vi "PrefDialog.vi"(8 "error in (no error)":errorcluster, 11 "MyPluginsBase in":refnum<class "NHRDCModel.lvclass">) -> (0 "error out":errorcluster, 1 "Save As":bool, 2 "Changed":bool, 3 "MyPluginsBase out":refnum<class "NHRDCModel.lvclass">)   [LabVIEW 2018, in "AcPwrPlugins.lvlib" / "NHRDCModel.lvclass"]
doc: "This VI displays the prior instruments properties and allows a user to change the instrument properties and save these new set properties to the same location on disk or in a new location with a new name called \"Type\"."
uses:
  NHRDCModel.lvclass
  <vilib>/Utility/config.llb/NI_LVConfig.lvlib
  AcPwrBaseClass/AcPwrBase.lvclass
  NHRDCPowerClass/TypeDefs/Modules.ctl
  NHRDCPowerClass/NHRDCPower.lvclass
  NHRDCPowerClass/TypeDefs/Device(s)Settings.ctl
  NHRDCPowerClass/TypeDefs/Measurements.ctl
panel:
  in  "btnSaveAs":bool
  in  "btnSave":bool
  in  "Measurement RefreshTime (ms)":u32
  in  "btnCancel":bool
  in  "Measurements":T1
  in  "Device(s)Settings":T2 {"Modules"."Regulation Gain (1=100%)" min=0.0 max=1.0; "Modules"."OutputSettings"."Wait on Value" items=["Voltage Greater Than Or Equal To", "Voltage Less Than Or Equal To", "Current Greater Than Or Equal To", "Current Less Than Or Equal To", "Power Greater Than Or Equal To", "Power Less Than Or Equal To"]; "Modules"."operating state (Off)" items=["Off", "Stand By", "Charge", "Discharge", "Battery Emulation"]}
  # "*Please ensure that Voltage and Current are selected as the 1st and 2nd Measurement variables, respectively, to correctly plot Voltage vs Current in the visualization VI."
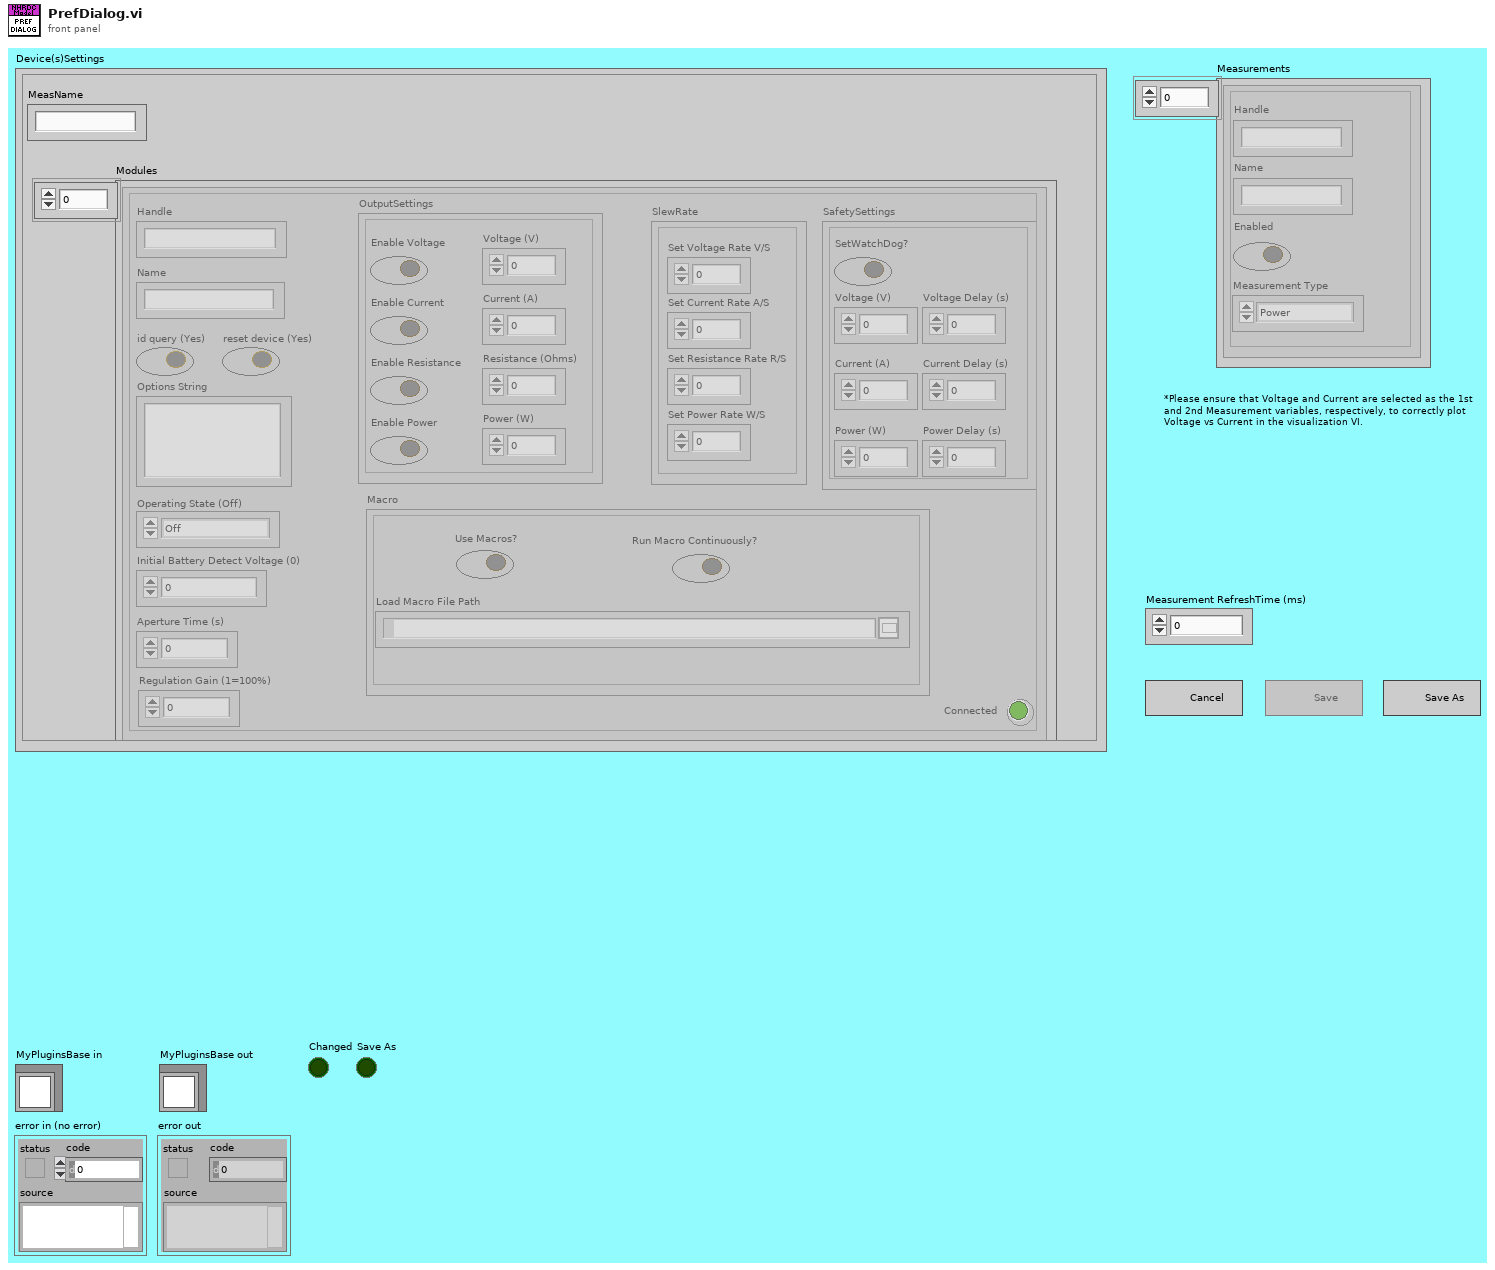
[diagram p1: front panel]
types:
  T1 = typedef "AcPwrPlugins.lvlib/NHRDCPower.lvclass/Measurements.ctl" = cluster{"Handle":string, "Name":string, "Enabled":bool, "Measurement Value":sgl, "Measurement Type":enum16{"Power", "Current", "Voltage"}}[]
  T2 = typedef "AcPwrPlugins.lvlib/NHRDCPower.lvclass/Device(s)Settings.ctl" = cluster{"MeasName":string, "Modules":T3}
  T3 = typedef "AcPwrPlugins.lvlib/NHRDCPower.lvclass/Modules.ctl" = cluster{"Handle":string, "Name":string, "id query (Yes)":bool, "reset device (Yes)":bool, "Connected":bool, "Initial Battery Detect Voltage (0)":dbl, "SafetySettings":cluster{"SetWatchDog?":bool, "Voltage (V)":dbl, "Current (A)":dbl, "Power (W)":dbl, "Voltage Delay (s)":dbl, "Current Delay (s)":dbl, "Power Delay (s)":dbl}, "Options String":string, "Aperture Time (s)":dbl, "operating state (Off)":i32, "OutputSettings":cluster{"Voltage (V)":dbl, "Current (A)":dbl, "Resistance (Ohms)":dbl, "Power (W)":dbl, "Enable Voltage":bool, "Enable Current":bool, "Enable Resistance":bool, "Enable Power":bool, "Macro After Step Delay  (s)":dbl, "Wait Value (V, A, W)":dbl, "Enable Wait":bool, "Wait on Value":i32}, "SlewRate":cluster{"Set Voltage Rate V/S":dbl, "Set Current Rate A/S":dbl, "Set Resistance Rate R/S":dbl, "Set Power Rate W/S":dbl}, "Macro":cluster{"Save Macro?":bool, "Load Macro From File?":bool, "Run Macro Continuously?":bool, "Use Macros?":bool, "Load Macro File Path":path, "Save Macro File Path":string}, "Regulation Gain (1=100%)":dbl, "UpdatingOntheFly":bool}[]
  T4 = enum8{"Enabled", "Disabled", "Disabled and Grayed Out"}
  T5 = enum32{"Invalid", "Default", "Floating", "Floating/Auto-Hide", "Modal"}
  T6 = cluster{"Handle":string, "Name":string, "id query (Yes)":bool, "reset device (Yes)":bool, "Connected":bool, "Initial Battery Detect Voltage (0)":dbl, "SafetySettings":cluster{"SetWatchDog?":bool, "Voltage (V)":dbl, "Current (A)":dbl, "Power (W)":dbl, "Voltage Delay (s)":dbl, "Current Delay (s)":dbl, "Power Delay (s)":dbl}, "Options String":string, "Aperture Time (s)":dbl, "operating state (Off)":i32, "OutputSettings":cluster{"Voltage (V)":dbl, "Current (A)":dbl, "Resistance (Ohms)":dbl, "Power (W)":dbl, "Enable Voltage":bool, "Enable Current":bool, "Enable Resistance":bool, "Enable Power":bool, "Macro After Step Delay  (s)":dbl, "Wait Value (V, A, W)":dbl, "Enable Wait":bool, "Wait on Value":i32}, "SlewRate":cluster{"Set Voltage Rate V/S":dbl, "Set Current Rate A/S":dbl, "Set Resistance Rate R/S":dbl, "Set Power Rate W/S":dbl}, "Macro":cluster{"Save Macro?":bool, "Load Macro From File?":bool, "Run Macro Continuously?":bool, "Use Macros?":bool, "Load Macro File Path":path, "Save Macro File Path":string}, "Regulation Gain (1=100%)":dbl, "UpdatingOntheFly":bool}
  T7 = typedef "AcPwrPlugins.lvlib/AcPwrBase.lvclass/BaseConfig.ctl" = cluster{"Frequency":dbl, "FrequencyRange":dbl[], "Phases":T8[], "Name":string, "PluginConfigVariant":variant, "PluginMeasVariant":variant}
  T8 = typedef "AcPwrPlugins.lvlib/AcPwrBase.lvclass/Phase.ctl" = cluster{"Name":string, "Enabled":bool, "VoltageLevel":dbl, "Handle":string, "VoltageRange":dbl[], "Connected":bool, "CurrentLimit":dbl, "Waveform":string}
  T9 = typedef "AcPwrPlugins.lvlib/AcPwrBase.lvclass/BaseMeasurements.ctl" = cluster{"Handle":string, "Name":string, "Enabled":bool, "Measurement Value":dbl, "btnMeasFetch":bool, "Chroma Hold Peak Current Measurement":bool, "Chroma Measurement Type":T10, "Chroma Protection Status String":string, "NHRDC Fetch Method":i32, "NHRDC Fetch Time (s)":sgl, "NHRDC Measurement Type":i32, "NHRGridSim Measurement Type ":enum16{"Average Current", "Max Current", "Min Current", "Average Voltage", "Max Voltage", "Min Voltage", "Average True Power", "Max True Power", "Min True Power", "Average Apparent Power", "Max Apparent Power", "Min Apparent Power", "Power Factor", "Crest Factor"}, "NHRGridSim Phase ":i32, "PPS Measurement Type ":enum16{"Voltage RMS L-N", "Voltage RMS L-L", "Frequency", "Current RMS", "Current Peak", "Crest Factor", "Power Factor", "Power VA", "Real Power"}, "PPS Channel Name":enum16{"A", "B", "C"}}[]
  T10 = typedef "AcPwrPlugins.lvlib/ChromaAcLoad.lvclass/MeasurementType.ctl" = enum16{"Voltage (Vrms or V)", "Current (Arms or A)", "Power (W)", "Peak Voltage (V)", "Peak Current (A)", "Peak Power (W)", "Frequency (Hz)", "Resistance (Ohms)", "Voltage Overshoot (V)", "Positive Peak Current (A)", "Voltage Undershoot (V)", "Negative Peak Current (A)", "Apparent Power (VA)", "Reacitive Power (VAR)", "Voltage THD", "Power Factor", "Current's Crest Factor"}
  T11 = typedef "NI_LVConfig.lvlib/Config Data RefNum.ctl" = refnum<k1>
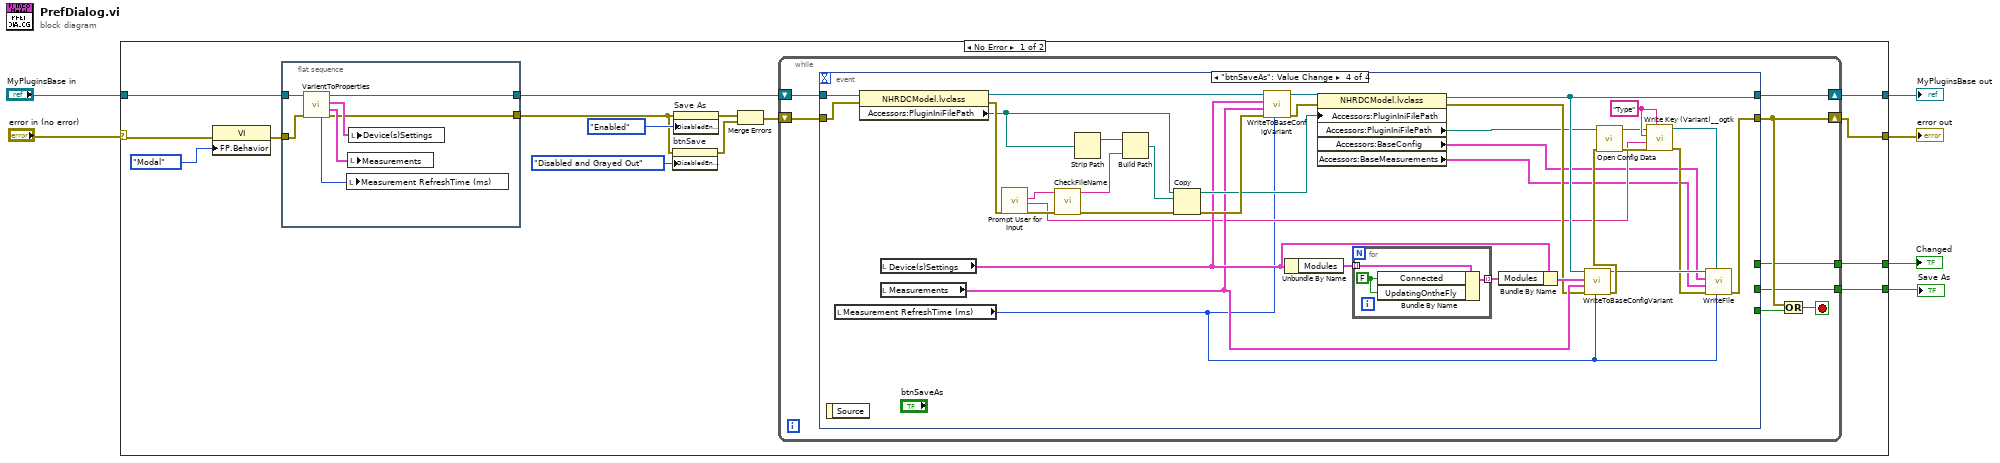
[diagram p0: block diagram]
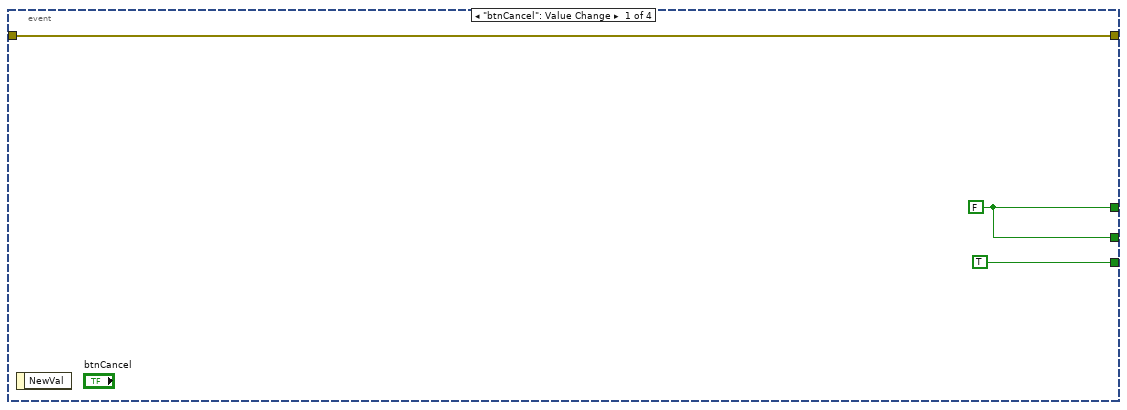
[diagram p2: hidden frame]
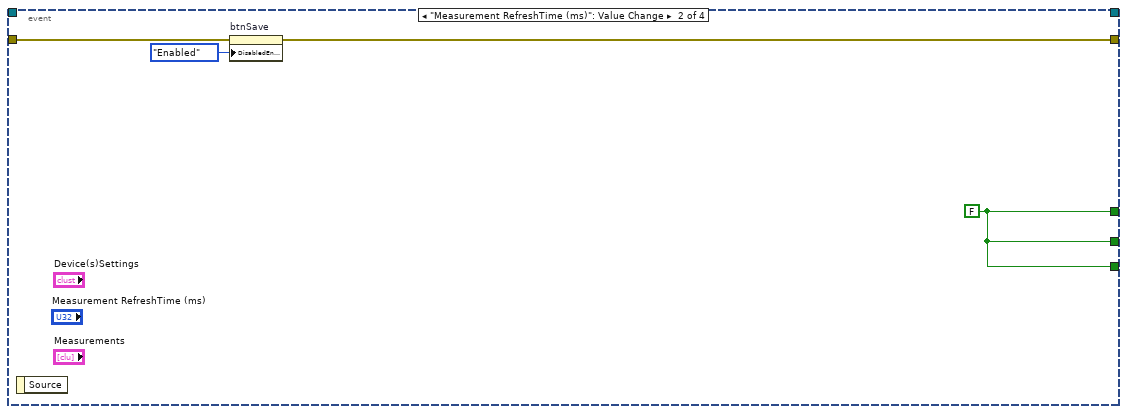
[diagram p3: hidden frame]
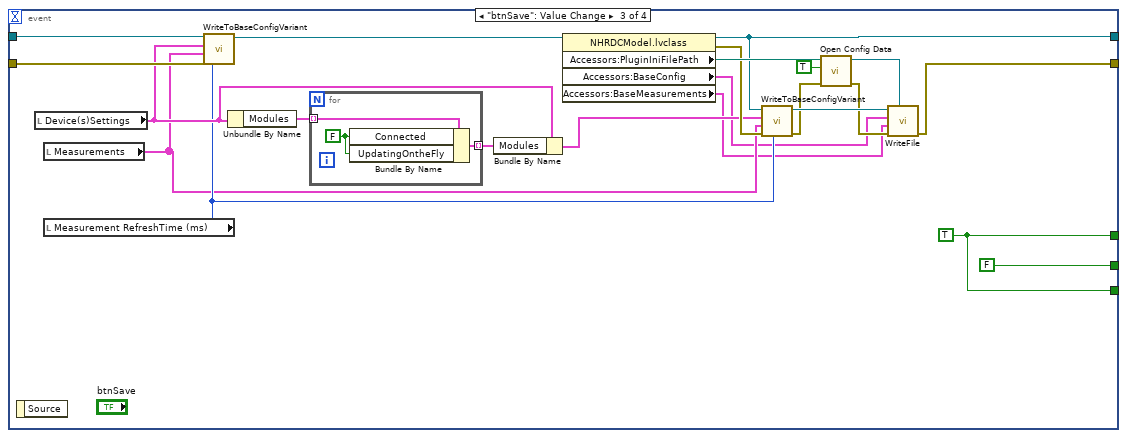
[diagram p4: hidden frame]
diagram:
  n1 = case shown="No Error" "error in (no error)" {
    selector: "error in (no error)" -> [w20 w107]
    tunnel: "MyPluginsBase in" -> [w19 w108]
    tunnel: [w10 w108] -> w4
    tunnel: [w9 w107] -> w3
    tunnel: [w8 _] -> w2
    tunnel: [w7 _] -> w1
    frame No Error {
      n2 = property class="VI"(error in=w20, "FP.Behavior"=T5."Modal" ("Front Panel Window:Behavior")) -> (error out=w18:errorcluster)  [unwired: 1 in, 1 out]
      n3 = flat-sequence {
        tunnel: w19 -> [w106]
        tunnel: w18 -> [w105]
        tunnel: [w101] -> w12
        tunnel: [w100] -> w16
        frame #0 {
          n4 = call "VarientToProperties.vi"("error in (no error)"=w105, "AcPwrPlugins.lvlib:NHRDCModel.lvclass"=w106) -> ("error out"=w100:errorcluster, "Measurements"=w103:T1, "Device(s)Settings"=w104:T2, "AcPwrPlugins.lvlib:NHRDCModel.lvclass"=w101:refnum<class "NHRDCModel.lvclass">, "Measurement Refresh Time (ms)"=w102:u32)  [unwired: 4 in, 1 out]
          n5 = local write "Measurement RefreshTime (ms)"(w102) -> ()
          n6 = local write "Measurements"(w103) -> ()
          n7 = local write "Device(s)Settings"(w104) -> ()
        }
      }
      n8 = property on="btnSave" class="Bool"(error in=w16, "DisabledEnum"=T4."Disabled and Grayed Out" ("Disabled")) -> (error out=w13:errorcluster)  [unwired: 1 in, 1 out]
      n9 = property on="Save As" class="Bool (strict)"(error in=w16, "DisabledEnum"=T4."Enabled" ("Disabled")) -> (error out=w14:errorcluster)  [unwired: 1 in, 1 out]
      n10 = Merge Errors(w14, w13) -> (w11:errorcluster)
      n11 = while {
        shift-right: [w24] -> w10
        shift-left: w12 -> [w29]
        shift-right: [w25] -> w9
        shift-left: w11 -> [w28]
        tunnel: [w23] -> w8
        tunnel: [w22] -> w7
        stop <- w26 stop-if-true
        n12 = event shown="[3] \"btnSaveAs\": Value Change" {
          selector: _ -> [_ _ _ _]
          dyn-events: _ -> [_ _ _ _]
          timeout: _ -> [_ _ _ _]
          tunnel: w29 -> [_ _ w58 w96]
          tunnel: w28 -> [w32 w36 w57 w95]
          tunnel: [w32 w34 w39 w65] -> w25
          tunnel: [TRUE w33 w37 _] -> w27
          tunnel: [w30 w33 w37 _] -> w23
          tunnel: [w30 w33 FALSE _] -> w22
          tunnel: [_ _ w50 w79] -> w24
          event "btnCancel": Value Change {
            w30 = FALSE
            n13 = event-data() -> ()  [unwired: 1 in, 1 out]
          }
          event "Measurement RefreshTime (ms)": Value Change {
            w33 = FALSE
            n14 = event-data() -> ()  [unwired: 1 in, 1 out]
            n15 = property on="btnSave" class="Bool"(error in=w36, "DisabledEnum"=T4."Enabled" ("Disabled")) -> (error out=w34:errorcluster)  [unwired: 1 in, 1 out]
          }
          event "btnSave": Value Change {
            w37 = TRUE
            n16 = event-data() -> ()  [unwired: 1 in, 1 out]
            n17 = local read "Device(s)Settings"() -> (w55:T2)
            n18 = local read "Measurements"() -> (w46:T1)
            n19 = local read "Measurement RefreshTime (ms)"() -> (w48:u32)
            n20 = call-dynamic "WriteToBaseConfigVariant.vi"("Measurement Refresh Time (ms)"=w48, "error in (no error)"=w57, "Meas"=w46, "Config"=w55, "NHRDCModel in"=w58) -> ("NHRDCModel out"=w53:refnum<class "NHRDCModel.lvclass">)  [unwired: 5 in, 1 out]
            n21 = Unbundle By Name(w55) -> ("Modules"=w56:T3)
            n22 = for {
              tunnel: w56 -> [w61] mode=indexing
              tunnel: [w59] -> w54 mode=indexing
              w60 = FALSE ("Connected")
              n23 = Bundle By Name(cluster=w61, "Connected"=w60, "UpdatingOntheFly"=w60) -> (w59:T6)
            }
            n24 = Bundle By Name(cluster=w55, "Modules"=w54) -> (w47:T2)
            n25 = property class="NHRDCModel.lvclass"(reference=w53) -> (reference out=w50:refnum<class "NHRDCModel.lvclass">, error out=w49:errorcluster, "Accessors:PluginIniFilePath"=w52:path, "Accessors:BaseConfig"=w41:T7, "Accessors:BaseMeasurements"=w40:T9)  [unwired: 1 in]
            n26 = call-dynamic "WriteToBaseConfigVariant.vi"("Measurement Refresh Time (ms)"=w48, "error in (no error)"=w49, "Meas"=w46, "Config"=w47, "NHRDCModel in"=w50) -> ("error out"=w44:errorcluster, "NHRDCModel out"=w45:refnum<class "NHRDCModel.lvclass">)  [unwired: 5 in]
            n27 = call <vilib>:"Open Config Data.vi"("error in (no error)"=w44, "create file if necessary (T)"=TRUE, "configuration file path"=w52) -> ("error out"=w43:errorcluster, "refnum"=w42:T11)  [unwired: 6 in, 1 out]
            n28 = call-dynamic "WriteFile.vi"("Refnum in"=w42, "error in (no error)"=w43, "BaseMeasurements"=w40, "BaseConfiguration"=w41, "NHRDCModel in"=w45) -> ("error out"=w39:errorcluster)  [unwired: 5 in, 1 out]
          }
          event "btnSaveAs": Value Change {
            w74 = "Type" ("section")
            n29 = event-data() -> ()  [unwired: 1 in, 1 out]
            n30 = local read "Measurement RefreshTime (ms)"() -> (w64:u32)
            n31 = property class="NHRDCModel.lvclass"(reference=w96, error in=w95) -> (reference out=w87:refnum<class "NHRDCModel.lvclass">, error out=w94:errorcluster, "Accessors:PluginIniFilePath"=w90:path)
            n32 = local read "Device(s)Settings"() -> (w80:T2)
            n33 = local read "Measurements"() -> (w77:T1)
            n34 = call "Prompt User for Input"("error in (no error)"=w94) -> ("File Name"=w70:string, "PluginType"=w69:string, "error out"=w93:errorcluster)  [unwired: 15 in, 1 out]
            n35 = call "CheckFileName.vi"("Error In"=w93, "File Name in"=w70) -> ("Error Out"=w88:errorcluster, "File Name out"=w91:string)  [unwired: 8 in]
            n36 = Strip Path(path=w90) -> (stripped path=w92:path)  [unwired: 1 out]
            n37 = Build Path(base path=w92, name or relative path=w91) -> (appended path=w89:path)
            n38 = Copy(8:w88, 10:w89, 11:w90) -> (0:w86:errorcluster, 3:w83:path)  [unwired: 2 in, 1 out]
            n39 = call-dynamic "WriteToBaseConfigVariant.vi"("Measurement Refresh Time (ms)"=w64, "error in (no error)"=w86, "Meas"=w77, "Config"=w80, "NHRDCModel in"=w87) -> ("error out"=w84:errorcluster, "NHRDCModel out"=w85:refnum<class "NHRDCModel.lvclass">)  [unwired: 5 in]
            n40 = Unbundle By Name(w80) -> ("Modules"=w82:T3)
            n41 = property class="NHRDCModel.lvclass"(reference=w85, error in=w84, "Accessors:PluginIniFilePath"=w83) -> (reference out=w79:refnum<class "NHRDCModel.lvclass">, error out=w76:errorcluster, "Accessors:PluginIniFilePath"=w75:path, "Accessors:BaseConfig"=w63:T7, "Accessors:BaseMeasurements"=w62:T9)
            n42 = for {
              tunnel: w82 -> [w99] mode=indexing
              tunnel: [w98] -> w81 mode=indexing
              w97 = FALSE ("Connected")
              n43 = Bundle By Name(cluster=w99, "Connected"=w97, "UpdatingOntheFly"=w97) -> (w98:T6)
            }
            n44 = Bundle By Name(cluster=w80, "Modules"=w81) -> (w78:T2)
            n45 = call-dynamic "WriteToBaseConfigVariant.vi"("Measurement Refresh Time (ms)"=w64, "error in (no error)"=w76, "Meas"=w77, "Config"=w78, "NHRDCModel in"=w79) -> ("error out"=w71:errorcluster, "NHRDCModel out"=w68:refnum<class "NHRDCModel.lvclass">)  [unwired: 5 in]
            n46 = call <vilib>:"Open Config Data.vi"("error in (no error)"=w71, "configuration file path"=w75) -> ("error out"=w72:errorcluster, "refnum"=w73:T11)  [unwired: 7 in, 1 out]
            n47 = call <userlib>:"Write Key (Variant)__ogtk.vi"("section"=w74, "error in (no error)"=w72, "key-value"=w69, "key (optional)"=w74, "refnum"=w73) -> ("error out"=w67:errorcluster, "refnum out"=w66:T11)  [unwired: 5 in]
            n48 = call-dynamic "WriteFile.vi"("RefreshTime"=w64, "Refnum in"=w66, "error in (no error)"=w67, "BaseMeasurements"=w62, "BaseConfiguration"=w63, "NHRDCModel in"=w68) -> ("error out"=w65:errorcluster)  [unwired: 4 in, 1 out]
          }
        }
        n49 = Or(x=w25, y=w27) -> (x .or. y?=w26:bool)
      }
    }
    frame Error {
    }
  }
  "error out" <- w3
  "MyPluginsBase out" <- w4
  "Save As" <- w1
  "Changed" <- w2
